vi "Periodic Tasks.vi"(8 "error in (no error)":errorcluster) -> ()   [LabVIEW 2014]
doc: "This VI runs in parallel to other tasks. It can contain as many user-defined periodic loops as you need. These can carry out PID or other sorts of timed response."
uses:
  Variables/References.vi
  Variables/Physical data.vi
  Variables/Default global.vi
  <vilib>/Rock Robotics/SystemInterfaces/Utilities/FPGA_UtilitiesRead LocalTime.vi
panel:
  in  "Pod number":i32
  in  "Iterations between saves":i32=1
  in  "General Configuration":T1
  out "All Pod State Data":T2(array[cluster])
  in  "Save":bool
  in  "PodConfigurations":T3(array[cluster])=[{"Drive"={"Encoder"={"CPft"=28.0, "Location"="TRT_SRX", "RIO_PinA"=0, "RIO_PinB"=0, "Invert?"=TRUE}, "Motor"={"PID"={"P"=1.0, "I"=1.0, "D"=1.0}, "CANorPWM Channel"=0, "Invert?"=FALSE, "IsCanSRX?"=FALSE, "Output"={"Max"=0.0, "Min"=0.0}}}, "Turret"={"Encoder"={"ZeroPosVolts"=4.313, "Location"="RIO", "RIO_AnalogChannel"=-4, "Invert?"=TRUE}, "Motor"={"PID"={"P"=1.0, "I"=1.0, "D"=1.0}, "CANorPWM Channel"=1, "Invert?"=FALSE, "IsCanSRX?"=TRUE, "Output"={"Max"=0.0, "Min"=0.0}}}, "Misc"={"Pod_Pos"={"X"=20.0, "Y"=34.0}, "PDP_Channels"={"Drive"=3, "Turret"=7}}}, {"Drive"={"Encoder"={"CPft"=25.0, "Location"="TRT_SRX", "RIO_PinA"=0, "RIO_PinB"=0, "Invert?"=TRUE}, "Motor"={"PID"={"P"=1.0, "I"=1.0, "D"=1.0}, "CANorPWM Channel"=1, "Invert?"=FALSE, "IsCanSRX?"=FALSE, "Output"={"Max"=0.0, "Min"=0.0}}}, "Turret"={"Encoder"={"ZeroPosVolts"=0.637, "Location"="RIO", "RIO_AnalogChannel"=1, "Invert?"=TRUE}, "Motor"={"PID"={"P"=1.0, "I"=1.0, "D"=-1.0}, "CANorPWM Channel"=2, "Invert?"=FALSE, "IsCanSRX?"=TRUE, "Output"={"Max"=0.0, "Min"=0.0}}}, "Misc"={"Pod_Pos"={"X"=4.0, "Y"=2.0}, "PDP_Channels"={"Drive"=10, "Turret"=11}}}, {"Drive"={"Encoder"={"CPft"=28.0, "Location"="TRT_SRX", "RIO_PinA"=0, "RIO_PinB"=0, "Invert?"=TRUE}, "Motor"={"PID"={"P"=1.0, "I"=1.0, "D"=1.0}, "CANorPWM Channel"=2, "Invert?"=FALSE, "IsCanSRX?"=FALSE, "Output"={"Max"=0.0, "Min"=0.0}}}, "Turret"={"Encoder"={"ZeroPosVolts"=3.14, "Location"="RIO", "RIO_AnalogChannel"=2, "Invert?"=FALSE}, "Motor"={"PID"={"P"=1.0, "I"=1.0, "D"=-6.0}, "CANorPWM Channel"=3, "Invert?"=FALSE, "IsCanSRX?"=TRUE, "Output"={"Max"=0.0, "Min"=0.0}}}, "Misc"={"Pod_Pos"={"X"=2.0, "Y"=32.0}, "PDP_Channels"={"Drive"=12, "Turret"=8}}}, {"Drive"={"Encoder"={"CPft"=28.0, "Location"="TRT_SRX", "RIO_PinA"=0, "RIO_PinB"=0, "Invert?"=TRUE}, "Motor"={"PID"={"P"=1.0, "I"=1.0, "D"=1.0}, "CANorPWM Channel"=3, "Invert?"=FALSE, "IsCanSRX?"=FALSE, "Output"={"Max"=0.0, "Min"=0.0}}}, "Turret"={"Encoder"={"ZeroPosVolts"=2.0, "Location"="RIO", "RIO_AnalogChannel"=3, "Invert?"=TRUE}, "Motor"={"PID"={"P"=1.0, "I"=1.0, "D"=10.0}, "CANorPWM Channel"=4, "Invert?"=FALSE, "IsCanSRX?"=TRUE, "Output"={"Max"=0.0, "Min"=0.0}}}, "Misc"={"Pod_Pos"={"X"=22.0, "Y"=4.0}, "PDP_Channels"={"Drive"=0, "Turret"=4}}}]
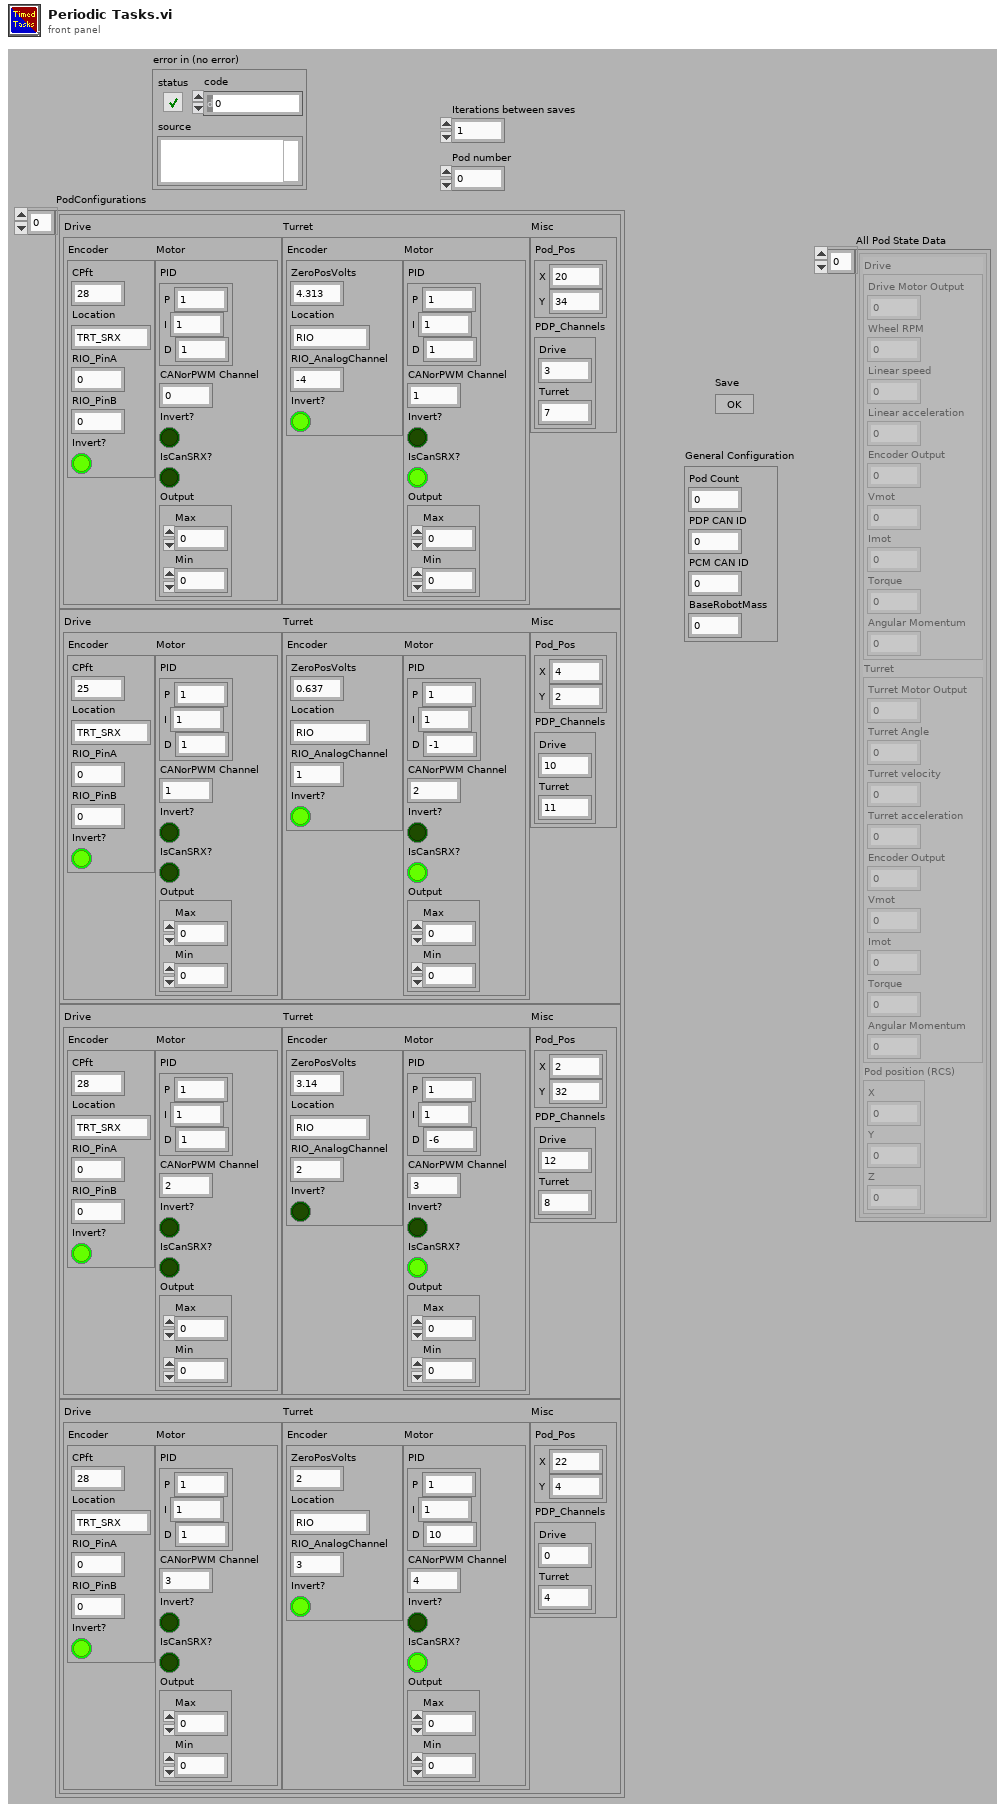
[diagram p1: front panel]
types:
  T1 = cluster{"Pod Count":i32, "PDP CAN ID":i32, "PCM CAN ID":i32, "BaseRobotMass":dbl}
  T2 = cluster{"Drive":cluster{"Drive Motor Output":dbl, "Wheel RPM":dbl, "Linear speed":dbl, "Linear acceleration":dbl, "Encoder Output":dbl, "Vmot":dbl, "Imot":dbl, "Torque":dbl, "Angular Momentum":dbl}, "Turret":cluster{"Turret Motor Output":dbl, "Turret Angle":dbl, "Turret velocity":dbl, "Turret acceleration":dbl, "Encoder Output":dbl, "Vmot":dbl, "Imot":dbl, "Torque":dbl, "Angular Momentum":dbl}, "Pod position (RCS)":cluster{"X":dbl, "Y":dbl, "Z":dbl}}[]
  T3 = cluster{"Drive":cluster{"Encoder":cluster{"CPft":dbl, "Location":string, "RIO_PinA":i32, "RIO_PinB":i32, "Invert?":bool}, "Motor":cluster{"PID":cluster{"P":dbl, "I":dbl, "D":dbl}, "CANorPWM Channel":i32, "Invert?":bool, "IsCanSRX?":bool, "Output":cluster{"Max":dbl, "Min":dbl}}}, "Turret":cluster{"Encoder":cluster{"ZeroPosVolts":dbl, "Location":string, "RIO_AnalogChannel":i32, "Invert?":bool}, "Motor":cluster{"PID":cluster{"P":dbl, "I":dbl, "D":dbl}, "CANorPWM Channel":i32, "Invert?":bool, "IsCanSRX?":bool, "Output":cluster{"Max":dbl, "Min":dbl}}}, "Misc":cluster{"Pod_Pos":cluster{"X":dbl, "Y":dbl}, "PDP_Channels":cluster{"Drive":i32, "Turret":i32}}}[]
  T4 = typedef "WPI_MotorControlDeviceRef.ctl" = cluster{"DeviceStatus":errorcluster, "Type":T5, "PWM":cluster{"Controller":T6, "PWM Channel":T7, "DeadBand":T8}, "CAN":cluster{"Device Number":u8, "Control Mode":T9, "Semaphore":T10, "Max Vout":dbl, "TalonSRX Control Mode":T11}, "Invert":bool, "TransformRef":T12, "InvTransformRef":T12}
  T5 = typedef "WPI_MotorControlType.ctl" = enum16{"PWM", "CAN", "CANTalonSRX"}
  T6 = typedef "FPGA_TypedefDigitalModule.ctl" = enum16{"Controller 1"}
  T7 = typedef "FPGA_DIOPWMChannel.ctl" = enum8{"PWM 0", "PWM 1", "PWM 2", "PWM 3", "PWM 4", "PWM 5", "PWM 6", "PWM 7", "PWM 8", "PWM 9", "PWM MXP 0", "PWM MXP 1", "PWM MXP 2", "PWM MXP 3", "PWM MXP 4", "PWM MXP 5", "PWM MXP 6", "PWM MXP 7", "PWM MXP 8", "PWM MXP 9", "Invalid"}
  T8 = typedef "WPI_PWMDeadband.ctl" = cluster{"Name":string, "maxPositivePwm":i32, "minPositivePwm":i32, "centerPwm":i32, "maxNegativePwm":i32, "minNegativePwm":i32, "angularRange":u16}
  T9 = typedef "WPI_CANJaguar_ControlMode.ctl" = enum8{"Percent VBus", "Current", "Speed", "Position", "Voltage"}
  T10 = typedef "Semaphore RefNum" = refnum<k1>
  T11 = typedef "WPI_CANTalonSRX_APIControlMode.ctl" = enum8{"Percent VBus", "Speed", "Position", "Slave", "Unchanged / Invalid"}
  T12 = typedef "WPI_PWMTransform_ConPane.ctl" = refnum<vi>
  T13 = typedef "WPI_AnalogChannelDevRef.ctl" = cluster{"DevStatus":errorcluster, "Controller":T14, "Analog Channel":T15}
  T14 = typedef "FPGA_TypedefAnalogModule.ctl" = enum16{"Controller 1"}
  T15 = typedef "FPGA_AIChannel.ctl" = enum8{"AI 0", "AI 1", "AI 2", "AI 3", "AI MXP 0", "AI MXP 1", "AI MXP 2", "AI MXP 3", "Invalid"}
  T16 = typedef "WPI_EncoderDevRef.ctl" = cluster{"DevStatus":errorcluster, "EncoderIndex":T17, "CounterIndex":T18, "DistancePerCount":dbl, "Decoding Type":T19}
  T17 = typedef "FPGA_EncoderIdx.ctl" = enum8{"Enc 0", "Enc 1", "Enc 2", "Enc 3", "Enc 4", "Enc 5", "Enc 6", "Enc 7", "Invalid"}
  T18 = typedef "FPGA_CounterCtrSystemIndex.ctl" = enum8{"Ctr 0", "Ctr 1", "Ctr 2", "Ctr 3", "Ctr 4", "Ctr 5", "Ctr 6", "Ctr 7", "Invalid"}
  T19 = typedef "WPI_EncoderType.ctl" = enum16{"1x", "2x", "4x"}
  T20 = cluster{"DriveMotorRef":T4, "TurretMotorRef":T4, "Turret Encoder":cluster{"AIDeviceRef":T13, "Turret Analog Location":enum16{"RoboRio", "Drive SRX", "Turret SRX"}}, "Drive Encoder":cluster{"EncoderDevRef":T16, "Drive Encoder Location":enum16{"RoboRio", "Drive SRX", "Turret SRX"}}, "Pod data":cluster{"Drive":cluster{"Encoder":cluster{"CPft":dbl, "Invert?":bool}, "Motor":cluster{"PID":cluster{"P":dbl, "I":dbl, "D":dbl}, "Invert?":bool, "IsCanSRX?":bool, "Output":cluster{"Max":dbl, "Min":dbl}}}, "Turret":cluster{"Encoder":cluster{"ZeroPosVolts":dbl, "Invert?":bool}, "Motor":cluster{"PID":cluster{"P":dbl, "I":dbl, "D":dbl}, "Invert?":bool, "IsCanSRX?":bool, "Output":cluster{"Max":dbl, "Min":dbl}}}, "Misc":cluster{"Pod_Pos":cluster{"X":dbl, "Y":dbl}, "PDP_Channels":cluster{"Drive":i32, "Turret":i32}}}, "Pod number":i32}[]
  T21 = cluster{"Sticks":cluster{"Left":cluster{"X":dbl, "Y":dbl, "Magnitude":dbl, "Direction":dbl, "Pressed?":bool}, "Right":cluster{"X":dbl, "Y":dbl, "Magnitude":dbl, "Direction":dbl, "Pressed?":bool}, "D-Pad":cluster{"X":dbl, "Y":dbl, "Directions":cluster{"North":bool, "Northeast":bool, "East":bool, "Southeast":bool, "South":bool, "Southwest":bool, "West":bool, "Northwest":bool}}}, "Buttons":cluster{"A":bool, "B":bool, "X":bool, "Y":bool, "L":bool, "R":bool, "Back":bool, "Start":bool}, "Triggers":cluster{"Left Trigger":cluster{"Depression":dbl, "Pressed":bool}, "Right Trigger":cluster{"Depression":dbl, "Pressed":bool}}, "Specials":cluster{"A \"SMASH\"":cluster{"Up":bool, "Down":bool, "Left":bool, "Right":bool}, "Double Tap":cluster{"A":bool, "B":bool, "X":bool, "Y":bool}, "Latching":cluster{"A":bool, "B":bool, "X":bool, "Y":bool, "L":bool, "R":bool, "Back":bool, "Start":bool}}}
  T22 = cluster{"DriveMotorRef":T4, "TurretMotorRef":T4, "Turret Encoder":cluster{"AIDeviceRef":T13, "Turret Analog Location":enum16{"RoboRio", "Drive SRX", "Turret SRX"}}, "Drive Encoder":cluster{"EncoderDevRef":T16, "Drive Encoder Location":enum16{"RoboRio", "Drive SRX", "Turret SRX"}}, "Pod data":cluster{"Drive":cluster{"Encoder":cluster{"CPft":dbl, "Invert?":bool}, "Motor":cluster{"PID":cluster{"P":dbl, "I":dbl, "D":dbl}, "Invert?":bool, "IsCanSRX?":bool, "Output":cluster{"Max":dbl, "Min":dbl}}}, "Turret":cluster{"Encoder":cluster{"ZeroPosVolts":dbl, "Invert?":bool}, "Motor":cluster{"PID":cluster{"P":dbl, "I":dbl, "D":dbl}, "Invert?":bool, "IsCanSRX?":bool, "Output":cluster{"Max":dbl, "Min":dbl}}}, "Misc":cluster{"Pod_Pos":cluster{"X":dbl, "Y":dbl}, "PDP_Channels":cluster{"Drive":i32, "Turret":i32}}}, "Pod number":i32}
  T23 = typedef "NI_LVConfig.lvlib/Config Data RefNum.ctl" = refnum<k1>
  T24 = typedef "NI_Matrix.lvlib/RealMatrix.ctl" = dbl[][]
  T25 = cluster{"All Pod State Data":cluster{"Drive":cluster{"Drive Motor Output":dbl, "Wheel RPM":dbl, "Linear speed":dbl, "Linear acceleration":dbl, "Encoder Output":dbl, "Vmot":dbl, "Imot":dbl, "Torque":dbl, "Angular Momentum":dbl}, "Turret":cluster{"Turret Motor Output":dbl, "Turret Angle":dbl, "Turret velocity":dbl, "Turret acceleration":dbl, "Encoder Output":dbl, "Vmot":dbl, "Imot":dbl, "Torque":dbl, "Angular Momentum":dbl}, "Pod position (RCS)":cluster{"X":dbl, "Y":dbl, "Z":dbl}}[], "Global Robot Data":cluster{"Position Data":cluster{"Robot Position":cluster{"X":dbl, "Y":dbl, "Z":dbl}, "Robot Velocity":cluster{"X":dbl, "Y":dbl, "Z":dbl}, "Robot Acceleration":cluster{"X":dbl, "Y":dbl, "Z":dbl}}, "Rotation Data":cluster{"Angular Position":cluster{"X":dbl, "Y":dbl, "Z":dbl}, "Angular Velocity":cluster{"X":dbl, "Y":dbl, "Z":dbl}, "Angular Acceleration":cluster{"X":dbl, "Y":dbl, "Z":dbl}}}, "Inertial Characteristics":cluster{"Center of Mass (RCS)":cluster{"X":dbl, "Y":dbl, "Z":dbl}, "Mass Elements":cluster{"X":dbl, "Y":dbl, "Z":dbl, "Mass":dbl, "Name":string}[], "Center of Rotation (RCS)":cluster{"X":dbl, "Y":dbl, "Z":dbl}, "Tensor of Inertia":T24}}
  T26 = cluster{"Position Data":cluster{"Robot Position":cluster{"X":dbl, "Y":dbl, "Z":dbl}, "Robot Velocity":cluster{"X":dbl, "Y":dbl, "Z":dbl}, "Robot Acceleration":cluster{"X":dbl, "Y":dbl, "Z":dbl}}, "Rotation Data":cluster{"Angular Position":cluster{"X":dbl, "Y":dbl, "Z":dbl}, "Angular Velocity":cluster{"X":dbl, "Y":dbl, "Z":dbl}, "Angular Acceleration":cluster{"X":dbl, "Y":dbl, "Z":dbl}}}
  T27 = cluster{"PodConfigurations":cluster{"Drive":cluster{"Encoder":cluster{"CPft":dbl, "Location":string, "RIO_PinA":i32, "RIO_PinB":i32, "Invert?":bool}, "Motor":cluster{"PID":cluster{"P":dbl, "I":dbl, "D":dbl}, "CANorPWM Channel":i32, "Invert?":bool, "IsCanSRX?":bool, "Output":cluster{"Max":dbl, "Min":dbl}}}, "Turret":cluster{"Encoder":cluster{"ZeroPosVolts":dbl, "Location":string, "RIO_AnalogChannel":i32, "Invert?":bool}, "Motor":cluster{"PID":cluster{"P":dbl, "I":dbl, "D":dbl}, "CANorPWM Channel":i32, "Invert?":bool, "IsCanSRX?":bool, "Output":cluster{"Max":dbl, "Min":dbl}}}, "Misc":cluster{"Pod_Pos":cluster{"X":dbl, "Y":dbl}, "PDP_Channels":cluster{"Drive":i32, "Turret":i32}}}[], "General Configuration":cluster{"Pod Count":i32, "PDP CAN ID":i32, "PCM CAN ID":i32, "BaseRobotMass":dbl}}
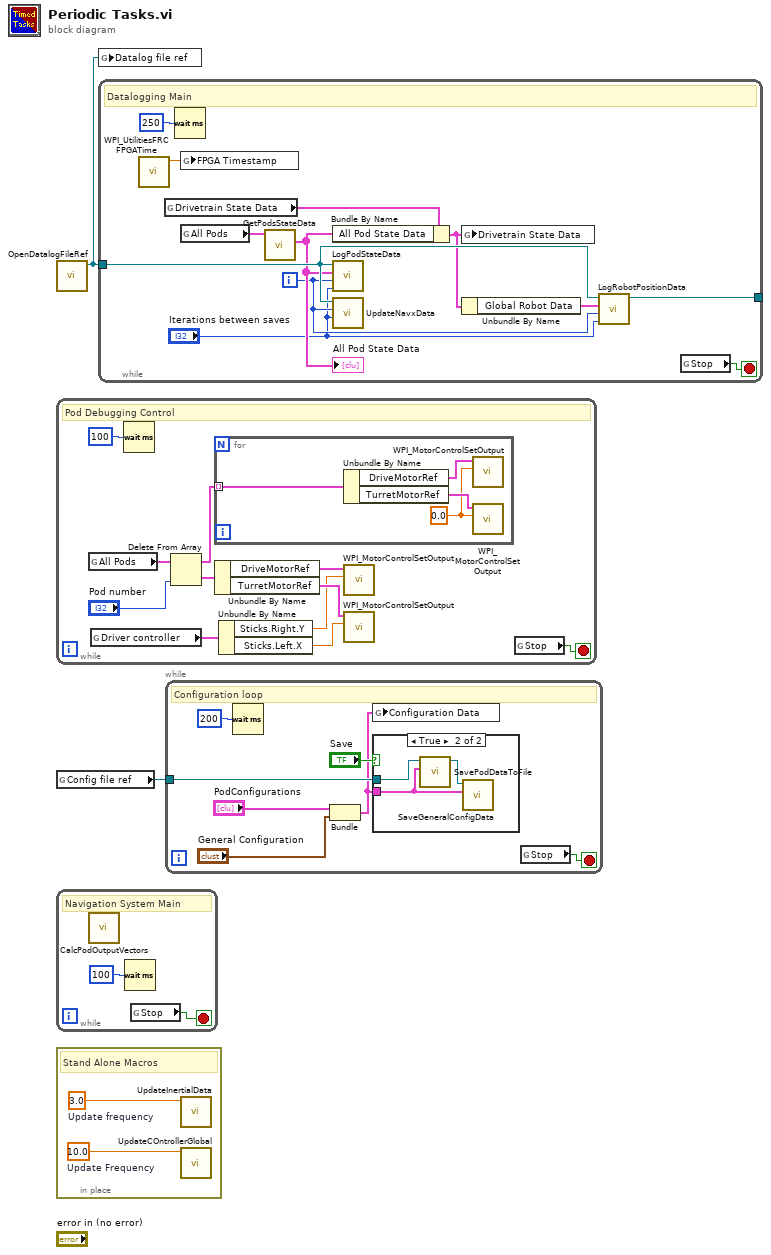
[diagram p0: block diagram]
diagram:
  n1 = call "OpenDatalogFileRef.vi"() -> ("tdms file out"=w1:refnum<k34>)  [unwired: 9 in, 2 out]
  n2 = while {
    stop <- w3 stop-if-true
    # "Pod Debugging Control"
    n3 = global read "References.vi" "All Pods"() -> (w13:T20)
    n4 = global read "Default global.vi" "Driver controller"() -> (w7:T21)
    n5 = Wait (ms)(milliseconds to wait=u32 100) -> ()  [unwired: 1 out]
    n6 = Delete From Array(array=w13, index="Pod number") -> (deleted portion=w10:T22, array with subset deleted=w11:T20)  [unwired: 1 in]
    n7 = for {
      tunnel: w11 -> [w17] mode=indexing
      w14 = 0.0 ("Output")
      n8 = Unbundle By Name(w17) -> ("DriveMotorRef"=w15:T4, "TurretMotorRef"=w16:T4)
      n9 = call <vilib>:"WPI_MotorControlSetOutput.vi"("Output"=w14, "MotorControlDevRef"=w15) -> ()  [unwired: 7 in, 3 out]
      n10 = call <vilib>:"WPI_MotorControlSetOutput.vi"("Output"=w14, "MotorControlDevRef"=w16) -> ()  [unwired: 7 in, 3 out]
    }
    n11 = Unbundle By Name(w10) -> ("DriveMotorRef"=w9:T4, "TurretMotorRef"=w8:T4)
    n12 = Unbundle By Name(w7) -> ("Sticks.Right.Y"=w6:dbl, "Sticks.Left.X"=w5:dbl)
    n13 = call <vilib>:"WPI_MotorControlSetOutput.vi"("Output"=w6, "MotorControlDevRef"=w9) -> ()  [unwired: 7 in, 3 out]
    n14 = call <vilib>:"WPI_MotorControlSetOutput.vi"("Output"=w5, "MotorControlDevRef"=w8) -> ()  [unwired: 7 in, 3 out]
    n15 = global read "Default global.vi" "Stop"() -> (w3:bool)
  }
  n16 = global read "References.vi" "Config file ref"() -> (w2:T23)
  n17 = while {
    stop <- w19 stop-if-true
    # "Navigation System Main"
    n18 = call "CalcPodOutputVectors.vi"() -> ()  [unwired: 11 in, 1 out]
    n19 = Wait (ms)(milliseconds to wait=u32 100) -> ()  [unwired: 1 out]
    n20 = global read "Default global.vi" "Stop"() -> (w19:bool)
  }
  n21 = in-place {
    w20 = 3.0  # Update frequency
    w21 = 10.0  # Update Frequency
    # "Stand Alone Macros"
    n22 = call "UpdateInertialData.vi"("Update frequency"=w20) -> ()  [unwired: 11 in]
    n23 = call "UpdateCOntrollerGlobal.vi"("Update Frequency"=w21) -> ()  [unwired: 11 in]
  }
  n24 = global write "References.vi" "Datalog file ref"(w1) -> ()
  n25 = while {
    tunnel: w1 -> [w28]
    tunnel: [w30] -> _
    i -> [w23]
    stop <- w24 stop-if-true
    # "Datalogging Main"
    n26 = call <vilib>:"WPI_UtilitiesFRC FPGATime.vi"() -> ("FPGA Time"=w31:dbl)  [unwired: 10 in, 1 out]
    n27 = global read "Physical data.vi" "Drivetrain State Data"() -> (w32:T25)
    n28 = Wait (ms)(milliseconds to wait=u32 250) -> ()  [unwired: 1 out]
    n29 = global write "Physical data.vi" "FPGA Timestamp"(w31) -> ()
    n30 = global read "References.vi" "All Pods"() -> (w29:T20)
    n31 = call "GetPodsStateData.vi"("All Pods In"=w29) -> ("All Pod State Data"=w25:T2)  [unwired: 9 in, 1 out]
    "All Pod State Data" <- w25
    n32 = Bundle By Name(cluster=w32, "All Pod State Data"=w25) -> (w27:T25)
    n33 = call "LogPodStateData.vi"("Iterations between saves"="Iterations between saves", "Iteration counter"=w23, "All Pod State Data"=w25, "Datalog File Refnum in"=w28) -> ()  [unwired: 7 in, 1 out]
    n34 = call "UpdateNavxData.vi"("Iterations between saves"="Iterations between saves", "Iteration counter"=w23, "Datalogging File Refnum in"=w28) -> ()  [unwired: 8 in, 1 out]
    n35 = global write "Physical data.vi" "Drivetrain State Data"(w27) -> ()
    n36 = Unbundle By Name(w27) -> ("Global Robot Data"=w26:T26)
    n37 = call "LogRobotPositionData.vi"("Iterations between saves"="Iterations between saves", "Iteration counter"=w23, "Global Robot Data"=w26, "Datalog File Refnum in"=w28) -> ("Datalog File Refnum out"=w30:refnum<k34>)  [unwired: 7 in]
    n38 = global read "Default global.vi" "Stop"() -> (w24:bool)
  }
  n39 = while {
    tunnel: w2 -> [w38]
    stop <- w35 stop-if-true
    # "Configuration loop"
    n40 = Wait (ms)(milliseconds to wait=u32 200) -> ()  [unwired: 1 out]
    n41 = Bundle("PodConfigurations"="PodConfigurations", "General Configuration"="General Configuration") -> (w34:T27)  [unwired: 1 in]
    n42 = global write "Physical data.vi" "Configuration Data"(w34) -> ()
    n43 = case shown="True" "Save" {
      tunnel: w38 -> [_ w43]
      tunnel: w34 -> [_ w41]
      frame False {
      }
      frame True {
        n44 = call "SavePodDataToFile.vi"("Configuration Data"=w41, "Config file Refnum in"=w43) -> ("Config file Refnum out"=w42:T23)  [unwired: 9 in]
        n45 = call "SaveGeneralConfigData.vi"("Configurations"=w41, "Refnum in"=w42) -> ()  [unwired: 9 in, 1 out]
      }
    }
    n46 = global read "Default global.vi" "Stop"() -> (w35:bool)
  }
